vi "Get Alarm Reason.vi"(8 "error in (no error)":errorcluster, 11 "Alarm in":refnum<class "Alarm.lvclass">) -> (0 "error out":errorcluster, 2 "Alarm Reason":string, 3 "Alarm out":refnum<class "Alarm.lvclass">)   [LabVIEW 2018, in "Alarm.lvclass"]
uses:
  Alarm.lvclass
  Alarm.lvclass/Alarm.ctl
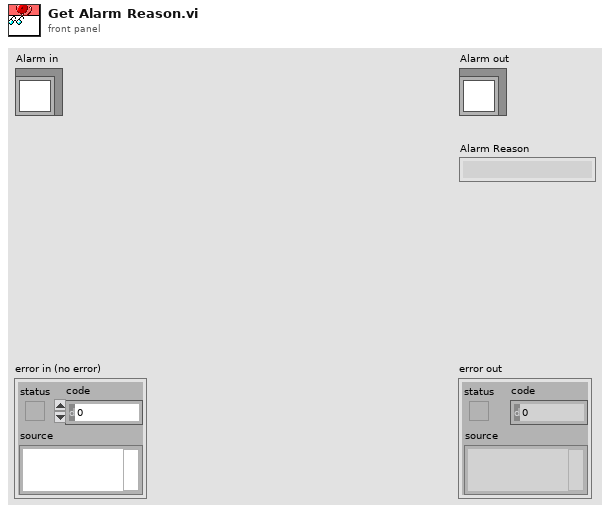
[diagram p1: front panel]
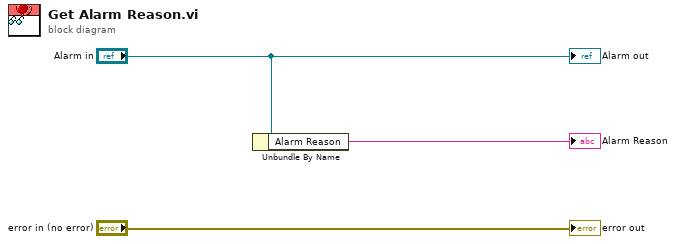
[diagram p0: block diagram]
diagram:
  n1 = Unbundle By Name("Alarm in") -> ("Alarm Reason"=→"Alarm Reason":string)
  "error out" <- "error in (no error)"
  "Alarm out" <- "Alarm in"
